vi "Unix Epoch to Timestamp.vi"(11 "String":string) -> (3 "Time Stamp":timestamp)   [LabVIEW 2026, in "TALOS.lvlib"]
uses:
  TALOS.lvlib
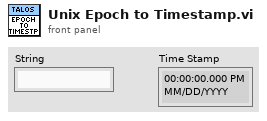
[diagram p1: front panel]
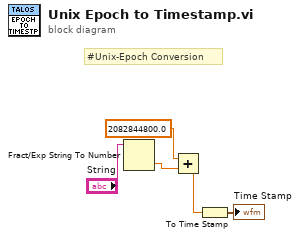
[diagram p0: block diagram]
diagram:
  # "#Unix-Epoch Conversion"
  n1 = Fract/Exp String To Number(string="String") -> (number=w2:dbl)  [unwired: 3 in, 1 out]
  n2 = Add(x=2082844800.0, y=w2) -> (x+y=w4:dbl)
  n3 = To Time Stamp(1:w4) -> (0:→"Time Stamp":timestamp)
